vi "SVFA Compensate Phase for Ref Frequencies (Complex) (1 Ch).vi"(0 "complex spectrum":T7={"complex spectrum response"={"f0"=0.0, "df"=1.0, "complex spectrum"=[]}, "spectrum info"={"channel name"="", "description"="", "x-axis units"=0, "spectral info"={"spectrum type"=enum."Power [Magnitude^2]", "linear/dB"=enum."linear", "window"=0, "window size"=0, "FFT size"=0}, "engineering units"=0, "custom label"="", "dB reference [EU]"=0.0, "peak units"=enum."rms", "weighting filter"=0, "spectral density?"=FALSE, "unit label"="", "spectrum skewed?"=FALSE, "complimentary spectrum units"=enum."none"}} {"spectrum info"."x-axis units" items=["Time (s)"=0, "Frequency-CB (Hz)"=1, "Frequency-CPB (Hz)"=1248, "Frequency-Arbitrary (Hz)"=2357, "Quefrency (s)"=2, "Revolutions (rev)"=3, "Order"=4, "Speed (RPM)"=11, "Speed (rad/s)"=21, "Index"=65535]; "spectrum info"."weighting filter" items=["Linear", "A-weighting", "B-weighting", "C-weighting", "ITU-R 468-4", "Dolby", "CCITT", "C-message", "Wb", "Wc", "Wd", "We", "Wf", "Wh", "Wj", "Wk", "Wm", "AES17 20 kHz lowpass", "AES17 40 kHz lowpass", "AES17 20 kHz highpass", "AES17 40 kHz highpass"]; "spectrum info"."dB reference [EU]" format="%.2f"; "spectrum info"."engineering units" items=["custom..."=0, "V"=1, "A"=21, "C"=30, "pC"=31, "s"=32, "-"=29, "Pa"=2, "N"=20, "g"=3, "m/s^2"=4, "m/s"=5, "m"=6, "mm/s"=12, "mm"=13, "micron/s"=14, "micron"=15, "in/s^2"=7, "in/s"=8, "in"=9, "mil/s"=10, "mil"=11, "rad/s^2"=16, "rad/s"=17, "rad"=18, "deg/s^2"=26, "deg/s"=27, "deg"=28, "RPM"=22, "cycle/s^2"=23, "Hz"=24, "cycle"=25, "strain"=19]; "spectrum info"."spectral info"."window" items=["None "=0, "Hanning"=1, "Hamming"=2, "Blackman-Harris"=3, "Exact Blackman"=4, "Blackman"=5, "Flat Top"=6, "4 Term B-Harris "=7, "7 Term B-Harris"=8, "Low Sidelobe"=9, "Force - Exponential"=10, "Gaussian"=62]; "complex spectrum response"."complex spectrum" format="%.2f"; "complex spectrum response"."df" format="%.2f"; "complex spectrum response"."f0" format="%.2f"}, 2 "reference frequencies [Hz]":dbl[](array[numeric]), 3 "advanced span [Hz]":dbl, 5 "error in":errorcluster) -> (14 "phase compensated complex spectrum":T7={"complex spectrum response"={"f0"=0.0, "df"=1.0, "complex spectrum"=[]}, "spectrum info"={"channel name"="", "description"="", "x-axis units"=0, "spectral info"={"spectrum type"=enum."Power [Magnitude^2]", "linear/dB"=enum."linear", "window"=0, "window size"=0, "FFT size"=0}, "engineering units"=0, "custom label"="", "dB reference [EU]"=0.0, "peak units"=enum."rms", "weighting filter"=0, "spectral density?"=FALSE, "unit label"="", "spectrum skewed?"=FALSE, "complimentary spectrum units"=enum."none"}} {"spectrum info"."x-axis units" items=["Time (s)"=0, "Frequency-CB (Hz)"=1, "Frequency-CPB (Hz)"=1248, "Frequency-Arbitrary (Hz)"=2357, "Quefrency (s)"=2, "Revolutions (rev)"=3, "Order"=4, "Speed (RPM)"=11, "Speed (rad/s)"=21, "Index"=65535]; "spectrum info"."weighting filter" items=["Linear", "A-weighting", "B-weighting", "C-weighting", "ITU-R 468-4", "Dolby", "CCITT", "C-message", "Wb", "Wc", "Wd", "We", "Wf", "Wh", "Wj", "Wk", "Wm", "AES17 20 kHz lowpass", "AES17 40 kHz lowpass", "AES17 20 kHz highpass", "AES17 40 kHz highpass"]; "spectrum info"."dB reference [EU]" format="%.2f"; "spectrum info"."engineering units" items=["custom..."=0, "V"=1, "A"=21, "C"=30, "pC"=31, "s"=32, "-"=29, "Pa"=2, "N"=20, "g"=3, "m/s^2"=4, "m/s"=5, "m"=6, "mm/s"=12, "mm"=13, "micron/s"=14, "micron"=15, "in/s^2"=7, "in/s"=8, "in"=9, "mil/s"=10, "mil"=11, "rad/s^2"=16, "rad/s"=17, "rad"=18, "deg/s^2"=26, "deg/s"=27, "deg"=28, "RPM"=22, "cycle/s^2"=23, "Hz"=24, "cycle"=25, "strain"=19]; "spectrum info"."spectral info"."window" items=["None "=0, "Hanning"=1, "Hamming"=2, "Blackman-Harris"=3, "Exact Blackman"=4, "Blackman"=5, "Flat Top"=6, "4 Term B-Harris "=7, "7 Term B-Harris"=8, "Low Sidelobe"=9, "Force - Exponential"=10, "Gaussian"=62]; "complex spectrum response"."complex spectrum" format="%.2f"; "complex spectrum response"."df" format="%.2f"; "complex spectrum response"."f0" format="%.2f"}, 19 "error out":errorcluster)   [LabVIEW 2017]
uses:
  <vilib>/addons/_NISVFA/_Shared subVIs/Controls/svc_Spectrum Info.ctl
  <vilib>/addons/_NISVFA/_Shared subVIs/Controls/svc_X-Axis Units.ctl
  <vilib>/addons/_NISVFA/_Shared subVIs/Controls/svc_Spectrum Type.ctl
  <vilib>/addons/_NISVFA/_Shared subVIs/Controls/svc_Engineering Units Text Ring.ctl
  <vilib>/addons/_NISVFA/_Shared subVIs/Controls/svc_Weighting Filter Text Ring.ctl
  <vilib>/addons/_NISVFA/_Shared subVIs/Controls/svc_Complimentary Spectrum Units.ctl
  <vilib>/addons/_NISVFA/_Spectrum Processing/SVFA Extract Multiple Tone Information (Complex) (1 Ch).vi
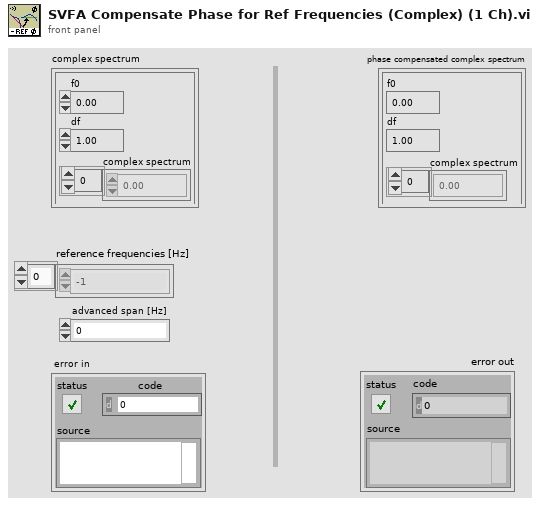
[diagram p1: front panel]
types:
  T1 = typedef "svc_Spectrum Info.ctl" = cluster{"channel name":string, "description":string, "x-axis units":T2, "spectral info":cluster{"spectrum type":T3, "linear/dB":enum16{"linear", "dB"}, "window":u16, "window size":i32, "FFT size":i32}, "engineering units":T4, "custom label":string, "dB reference [EU]":dbl, "peak units":enum16{"rms", "peak", "peak-peak"}, "weighting filter":T5, "spectral density?":bool, "unit label":string, "spectrum skewed?":bool, "complimentary spectrum units":T6}
  T2 = typedef "svc_X-Axis Units.ctl" = u16
  T3 = typedef "svc_Spectrum Type.ctl" = enum16{"FFT Spectrum [complex]", "Amplitude [Magnitude]", "Power [Magnitude^2]", "Cross Spectrum [complex]", "Frequency Response [Complex]"}
  T4 = typedef "svc_Engineering Units Text Ring.ctl" = u16
  T5 = typedef "svc_Weighting Filter Text Ring.ctl" = u16
  T6 = typedef "svc_Complimentary Spectrum Units.ctl" = enum16{"none", "radians", "degrees", "cycles", "imaginary"}
  T7 = cluster{"complex spectrum response":cluster{"f0":dbl, "df":dbl, "complex spectrum":cdb[]}, "spectrum info":T1}
  T8 = enum32{"none", "input signal", "detected signal", "residual signal"}
  T9 = cluster{"frequency [Hz]":dbl, "amplitude [EU pk]":dbl, "phase (deg)":dbl}[]
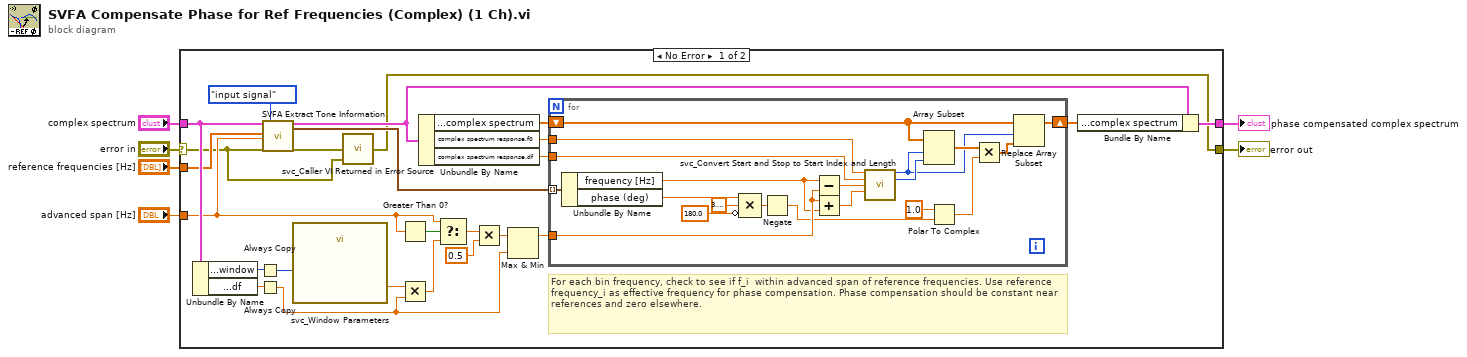
[diagram p0: block diagram]
diagram:
  n1 = case shown="No Error" "error in" {
    selector: "error in" -> [w7 w53]
    tunnel: "complex spectrum" -> [w29 w52]
    tunnel: "advanced span [Hz]" -> [w11 _]
    tunnel: "reference frequencies [Hz]" -> [w28 _]
    tunnel: [w8 w53] -> w3
    tunnel: [w25 w52] -> w1
    frame No Error {
      # "For each bin frequency, check to see if f_i  within advanced span of reference frequencies. Use reference frequency_i as effective frequency for phase compensation. Phase compensation should be constant near references and zero elsewhere."
      n2 = Unbundle By Name(w29) -> ("spectrum info.spectral info.window"=w31:u16, "complex spectrum response.df"=w27:dbl)
      n3 = Always Copy(1:w31) -> (0:w30:u16)
      n4 = Always Copy(1:w27) -> (0:w26:dbl)
      n5 = call-poly <vilib>:"SVFA Extract Tone Information.vi"("complex spectrum"=w29, "expected frequencies [Hz]"=w28, "advanced span [Hz]"=w11, "error in"=w7, "export signals"=T8."input signal") -> ("complex spectrum"=w13:T7, "detected tones"=w12:T9, "error out"=w9:errorcluster)  [unwired: 11 in, 1 out]
      n6 = call <vilib>:"svc_Window Parameters.vi"("window"=w30) -> ("maximum BW"=w23:dbl)  [unwired: 7 in, 3 out]
      n7 = call <vilib>:"svc_Caller VI Returned in Error Source.vi"("warning input to caller"=w7, "error in (no error)"=w9) -> ("error out"=w8:errorcluster)  [unwired: 3 in]
      n8 = Greater Than 0?(x=w11) -> (x > 0?=w24:bool)
      n9 = Multiply(x=w23, y=w26) -> (x*y=w22:dbl)
      n10 = Unbundle By Name(w13) -> ("complex spectrum response.complex spectrum"=w18:cdb[], "complex spectrum response.f0"=w17:dbl, "complex spectrum response.df"=w16:dbl)
      n11 = Select(t=w11, s=w24, f=w22) -> (s? t:f=w20:dbl)
      n12 = Multiply(x=w20, y=0.5 ("value")) -> (x*y=w19:dbl)
      n13 = Max & Min(x=w19, y=w26) -> (max(x,y)=w15:dbl)  [unwired: 1 out]
      n14 = for {
        tunnel: w17 -> [w41]
        tunnel: w16 -> [w40]
        tunnel: w15 -> [w51]
        shift-right: [w35] -> w14
        shift-left: w18 -> [w38]
        tunnel: w12 -> [w45] mode=indexing
        n15 = Unbundle By Name(w45) -> ("frequency [Hz]"=w44:dbl, "phase (deg)"=w33:dbl)
        n16 = Compound Arithmetic op=MULTIPLY(w33, 3.141592653589793 ("x"), invert 180.0 ("y")) -> (w48:dbl)
        n17 = Negate(x=w48) -> (-x=w32:dbl)
        n18 = Subtract(x=w44, y=w51) -> (x-y=w42:dbl)
        n19 = Add(x=w51, y=w44) -> (x+y=w43:dbl)
        n20 = call <vilib>:"svc_Convert Start and Stop to Start Index and Length.vi"("f0"=w41, "df"=w40, "start frequency"=w42, "stop frequency"=w43) -> ("start index"=w34:i32, "band length"=w39:i32)  [unwired: 8 in, 2 out]
        n21 = Array Subset(array=w38, index=w34, length=w39) -> (w37:cdb[])
        n22 = Polar To Complex(1:w32, 2:1.0 ("x")) -> (0:w49:cdb)
        n23 = Multiply(x=w37, y=w49) -> (x*y=w36:cdb[])
        n24 = Replace Array Subset(array=w38, new element=w36, index=w34) -> (w35:cdb[])
      }
      n25 = Bundle By Name(cluster=w13, "complex spectrum response.complex spectrum"=w14) -> (w25:T7)
    }
    frame Error {
    }
  }
  "phase compensated complex spectrum" <- w1
  "error out" <- w3
